vi "CreateZip.vi"(6 "Source Dir":path, 7 "Destination Directory":path, 11 "ZIP File Name":string) -> ()   [LabVIEW 2014]
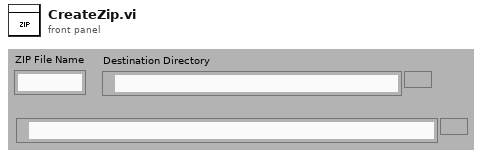
[diagram p1: front panel]
types:
  T1 = enum16{"open", "replace", "create", "open or create", "replace or create", "replace or create with confirmation"}
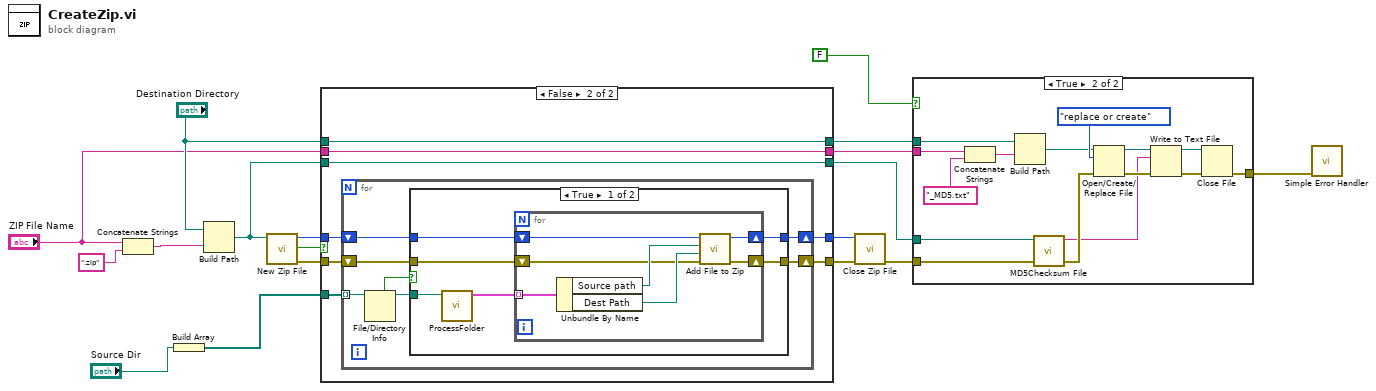
[diagram p0: block diagram]
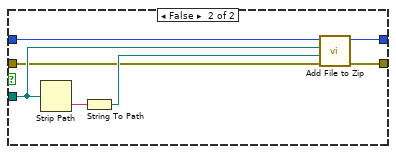
[diagram p4: hidden frame]
diagram:
  n1 = Concatenate Strings("ZIP File Name", ".zip" ("string")) -> (w4:string)
  n2 = Build Array("Source Dir") -> (w1:path[])
  n3 = Build Path(base path="Destination Directory", name or relative path=w4) -> (appended path=w13:path)
  n4 = call <vilib>:"New Zip File.vi"("target"=w13) -> ("error out"=w15:errorcluster, "cancelled"=w18:bool, "zip file out"=w17:i64)  [unwired: 4 in]
  n5 = case shown="False" w18 {
    tunnel: w17 -> [w23 w30]
    tunnel: w1 -> [_ w31]
    tunnel: [w23 w29] -> w16
    tunnel: w15 -> [w22 w28]
    tunnel: [w22 w27] -> w14
    tunnel: w13 -> [w21 w26]
    tunnel: [w21 w26] -> w12
    tunnel: "Destination Directory" -> [w20 w25]
    tunnel: [w20 w25] -> w9
    tunnel: "ZIP File Name" -> [w19 w24]
    tunnel: [w19 w24] -> w7
    frame True {
    }
    frame False {
      n6 = for {
        tunnel: w31 -> [w36] mode=indexing
        shift-right: [w37] -> w29
        shift-left: w30 -> [w38]
        shift-right: [w32] -> w27
        shift-left: w28 -> [w33]
        n7 = File/Directory Info(path=w36) -> (path out=w35:path, directory=w34:bool)  [unwired: 1 in, 5 out]
        n8 = case shown="True" w34 {
          tunnel: w38 -> [w42 w58]
          tunnel: [w41 w57] -> w37
          tunnel: w35 -> [w44 w54]
          tunnel: w33 -> [w40 w53]
          tunnel: [w39 w52] -> w32
          frame True {
            n9 = call "ProcessFolder.vi"("Path"=w44) -> ("Array"=w43:cluster{"Source path":path, "Dest Path":path}[])  [unwired: 10 in]
            n10 = for {
              tunnel: w43 -> [w51] mode=indexing
              shift-right: [w49] -> w41
              shift-left: w42 -> [w50]
              shift-right: [w45] -> w39
              shift-left: w40 -> [w46]
              n11 = Unbundle By Name(w51) -> ("Source path"=w48:path, "Dest Path"=w47:path)
              n12 = call <vilib>:"Add File to Zip.vi"("error in (no error)"=w46, "destination path in zip"=w47, "source file path"=w48, "zip file in"=w50) -> ("error out"=w45:errorcluster, "zip file out"=w49:i64)  [unwired: 6 in]
            }
          }
          frame False {
            n13 = Strip Path(path=w54) -> (name=w56:string)  [unwired: 1 out]
            n14 = String To Path(string=w56) -> (path=w55:path)
            n15 = call <vilib>:"Add File to Zip.vi"("error in (no error)"=w53, "destination path in zip"=w55, "source file path"=w54, "zip file in"=w58) -> ("error out"=w52:errorcluster, "zip file out"=w57:i64)  [unwired: 6 in]
          }
        }
      }
    }
  }
  n16 = call <vilib>:"Close Zip File.vi"("error in (no error)"=w14, "zip file in"=w16) -> ("error out"=w11:errorcluster)  [unwired: 5 in]
  n17 = case shown="True" FALSE {
    tunnel: w12 -> [_ w74]
    tunnel: w11 -> [w59 w73]
    tunnel: w9 -> [_ w64]
    tunnel: [w59 w65] -> w8
    tunnel: w7 -> [_ w62]
    frame False {
    }
    frame True {
      n18 = Concatenate Strings(w62, "_MD5.txt" ("name or relative path")) -> (w60:string)
      n19 = Build Path(base path=w64, name or relative path=w60) -> (appended path=w63:path)
      n20 = call <vilib>:"MD5Checksum File.vi"("error in (no error)"=w73, "Path"=w74) -> ("error out"=w72:errorcluster, "MD5 message-digest"=w69:string)  [unwired: 8 in]
      n21 = Open/Create/Replace File(file path (use dialog)=w63, error in=w72, operation (0:open)=T1."replace or create") -> (refnum out=w68:refnum<file>, error out=w70:errorcluster)  [unwired: 3 in, 1 out]
      n22 = Write to Text File(file (use dialog)=w68, text=w69, error in=w70) -> (refnum out=w66:refnum<file>, error out=w67:errorcluster)  [unwired: 1 in, 1 out]
      n23 = Close File(refnum=w66, error in=w67) -> (error out=w65:errorcluster)  [unwired: 1 out]
    }
  }
  n24 = call <vilib>:"Simple Error Handler.vi"("error in (no error)"=w8) -> ()  [unwired: 4 in, 5 out]
